vi "motor control proto.vi"(4 "minimal rot error":dbl=0.001, 6 "minimal error":dbl=0.001, 7 "motor link":enum16{"平移", "旋转", "压电控制"}(ring), 8 "error in (no error)":errorcluster caption="错误输入（无错误）", 9 "rotation num":dbl, 10 "target position":dbl=0.2 min=0.2 max=25.0 step=0.002) -> (0 "error out":errorcluster caption="错误输出", 1 "rotaion":dbl, 2 "position":dbl)   [LabVIEW 2017]
doc: "该模板用于创建子VI。"
uses:
  motor control.ctl
panel:
  out "Position":dbl[](array[numeric]) format="%.6f"
  in  "obj error":dbl=0.001
  out "objective":dbl min=0.0 max=250.0
  in  "target objective":dbl min=0.0 max=250.0
  in  "USB SET for E709":cluster{"S/N":string, "USB Search?":bool}={"S/N"="", "USB Search?"=TRUE}
  in  "RON settings 2":T1={"RON Affected axes"=[], "Reference mode"=[], "Check FRF?"=TRUE}
  in  "RON settings":T1={"RON Affected axes"=[], "Reference mode"=[], "Check FRF?"=TRUE}
  in  "DaisyChain settings for rotation":T2={"Register DC"=FALSE, "DaisyChain Search?"=TRUE, "Device ID"=2}
  in  "USB settings for rotation":cluster{"S/N":string, "USB Search?":bool}={"S/N"="0135500392", "USB Search?"=FALSE}
  in  "DaisyChain setting for move":T2={"Register DC"=FALSE, "DaisyChain Search?"=TRUE, "Device ID"=1}
  in  "USB setting for move":cluster{"S/N":string, "USB Search?":bool}={"S/N"="0135500392", "USB Search?"=FALSE}
  in  "断开通讯":bool
  in  "motor control":T3={"System no."=1, "Conn. \nAxes"=[], "当前数值"=[]} {"System no." min=1 step=1}
  # "parameter set"
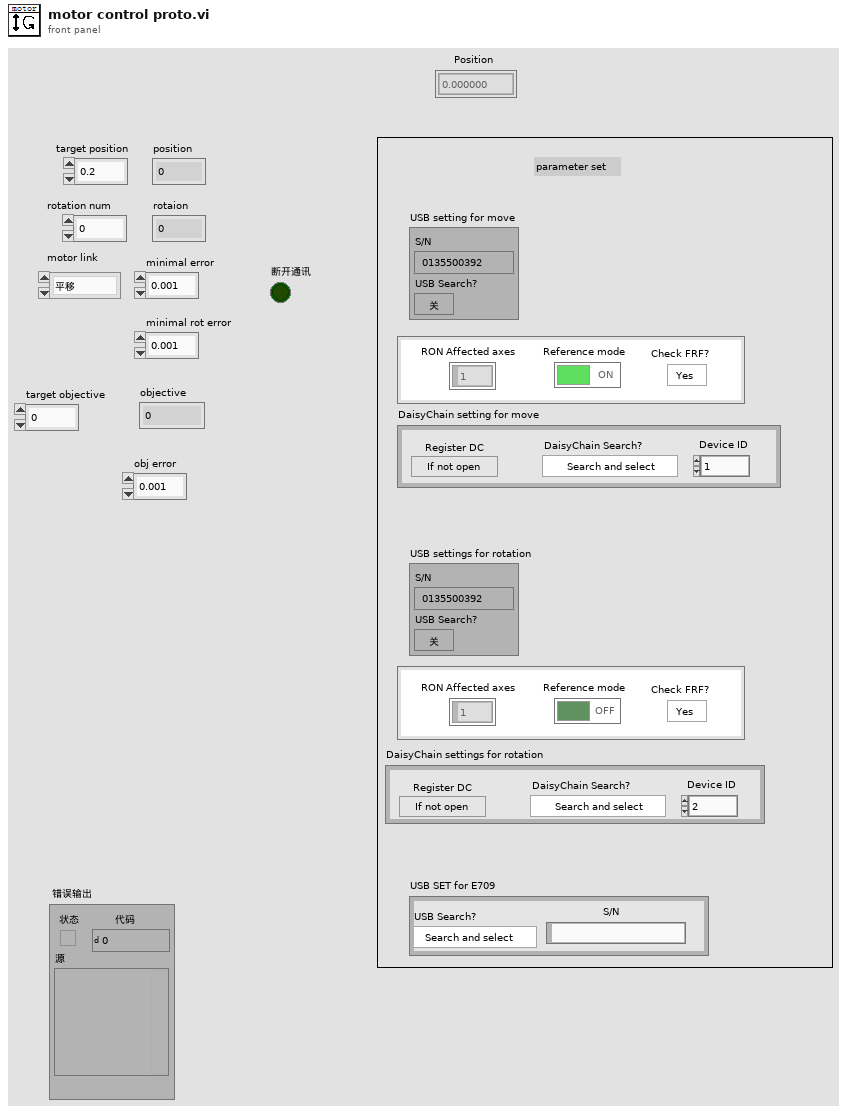
[diagram p1: front panel]
types:
  T1 = cluster{"RON Affected axes":string[], "Reference mode":bool[], "Check FRF?":bool}
  T2 = cluster{"Register DC":bool, "DaisyChain Search?":bool, "Device ID":i32}
  T3 = typedef "motor control.ctl" = cluster{"System no.":i32, "Conn. \nAxes":string[], "当前数值":dbl[]}
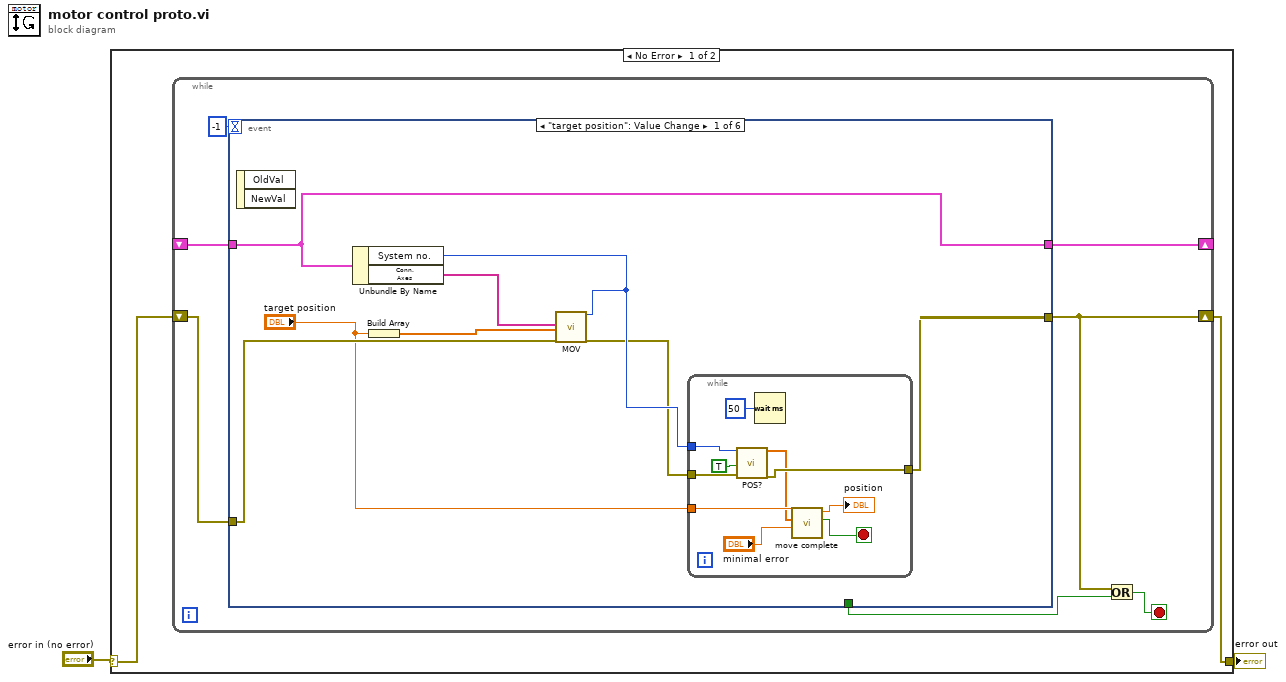
[diagram p0: block diagram]
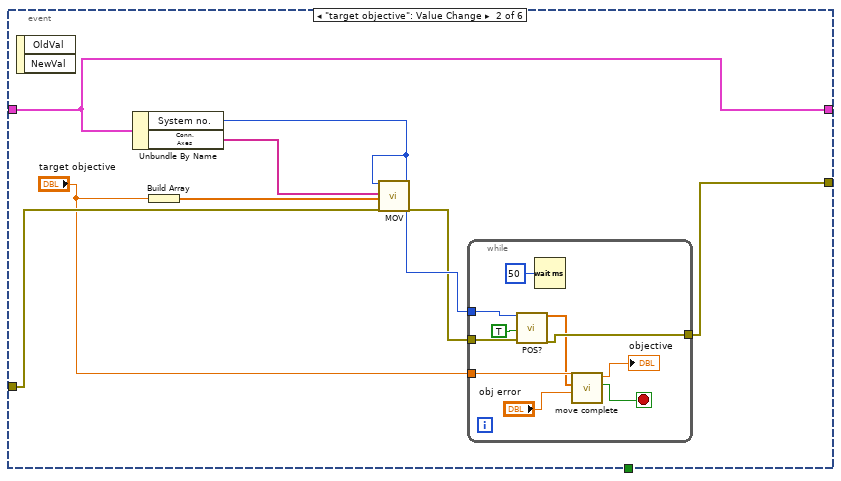
[diagram p2: hidden frame]
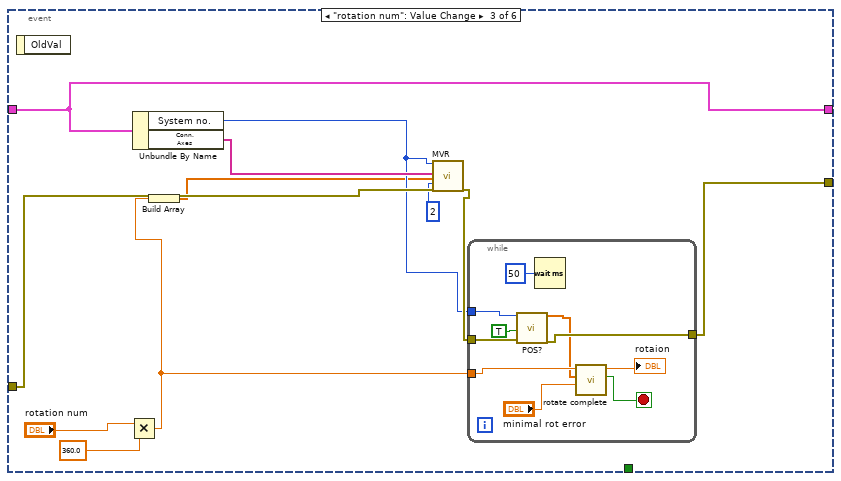
[diagram p3: hidden frame]
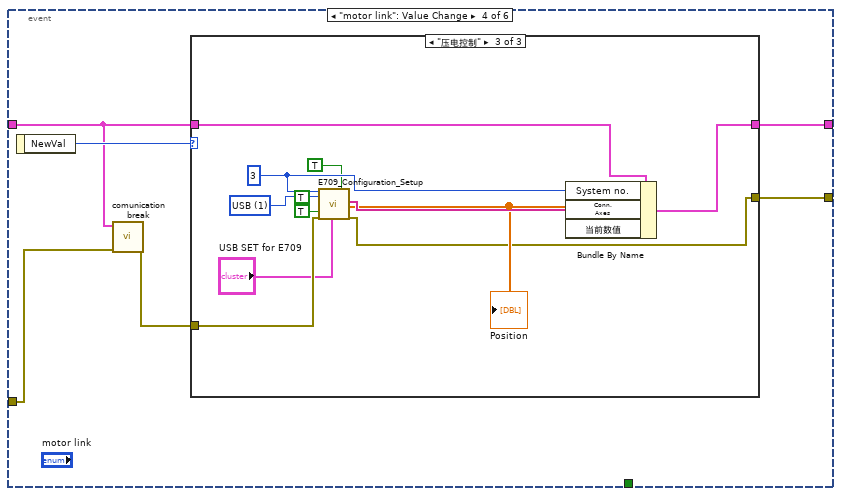
[diagram p4: hidden frame]
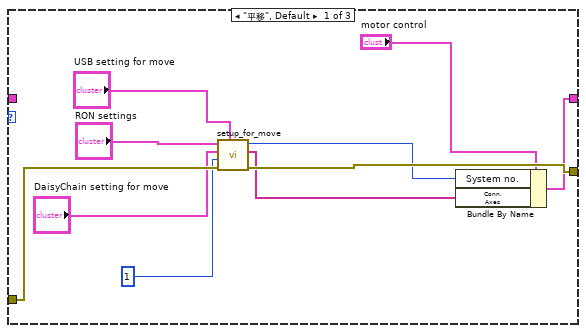
[diagram p5: hidden frame]
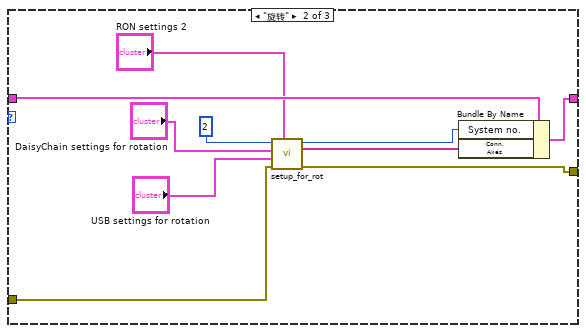
[diagram p6: hidden frame]
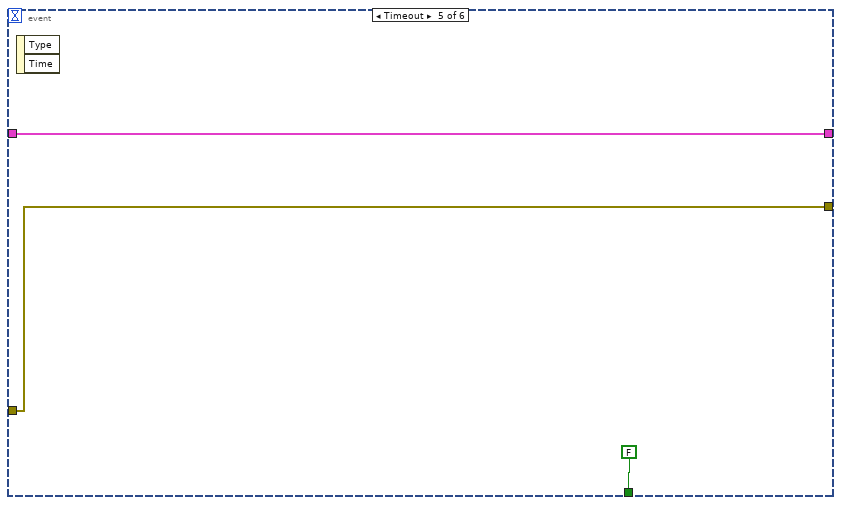
[diagram p7: hidden frame]
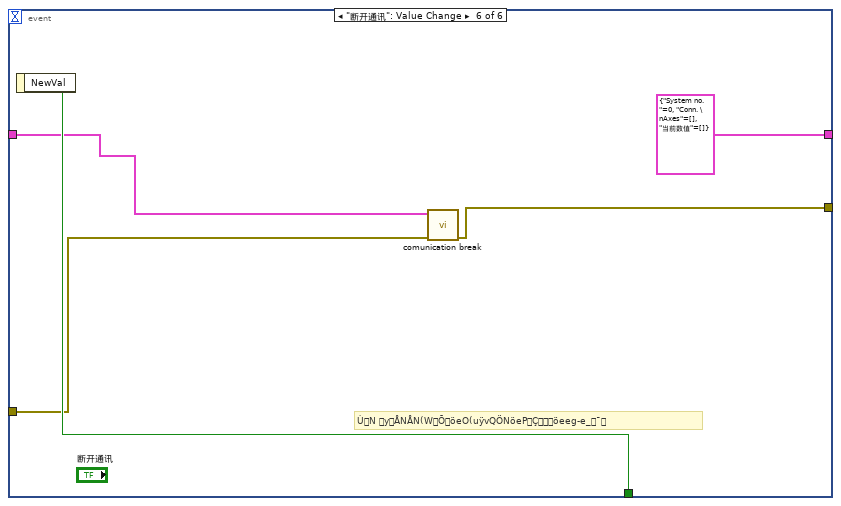
[diagram p8: hidden frame]
diagram:
  n1 = case shown="No Error" "error in (no error)" {
    selector: "error in (no error)" -> [w3 w115]
    tunnel: [w4 w115] -> w1
    frame No Error {
      n2 = while {
        shift-right: [w6] -> w4
        shift-left: w3 -> [w9]
        shift-right: [w11] -> _
        shift-left: _ -> [w10]
        stop <- w5 stop-if-true
        n3 = event shown="[0] \"target position\": Value Change" {
          selector: _ -> [_ _ _ _ _ _]
          dyn-events: _ -> [_ _ _ _ _ _]
          timeout: -1 -> [_ _ _ _ _ _]
          tunnel: [w13 w31 w57 w74 w107 w111] -> w6
          tunnel: w9 -> [w18 w36 w53 w71 w107 w112]
          tunnel: [w17 w35 w58 w73 w109 T3 {"System no."=0, "Conn. \nAxes"=[], "当前数值"=[]} ("motor control 2")] -> w11
          tunnel: w10 -> [w17 w35 w58 w69 w109 w113]
          tunnel: [_ _ _ _ FALSE ("NewVal") w114] -> w7
          event "target position": Value Change {
            n4 = event-data() -> ()  [unwired: 1 in, 2 out]
            n5 = Unbundle By Name(w17) -> ("System no."=w16:i32, "Conn. \nAxes"=w19:string[])
            n6 = Build Array("target position") -> (w14:dbl[])
            n7 = call "MOV.vi"("System no."=w16, "Axes to move"=w19, "Position values"=w14, "error in"=w18) -> ("error out"=w15:errorcluster)  [unwired: 15 in]
            n8 = while {
              tunnel: w16 -> [w29]
              tunnel: w15 -> [w27]
              tunnel: [w26] -> w13
              tunnel: "target position" -> [w23]
              stop <- w20 stop-if-true
              n9 = call "POS?.vi"("System no."=w29, "All axes?"=TRUE, "error in"=w27) -> ("Position"=w22:dbl[], "error out"=w26:errorcluster)  [unwired: 15 in]
              n10 = Wait (ms)(milliseconds to wait=u32 50 ("等待时间（毫秒）")) -> ()  [unwired: 1 out]
              n11 = call "move complete.vi"("minimal error"="minimal error", "Position"=w22, "target position"=w23) -> (2:w20:bool, "position output"=→"position":dbl)  [unwired: 6 in, 1 out]
            }
          }
          event "target objective": Value Change {
            n12 = event-data() -> ()  [unwired: 1 in, 2 out]
            n13 = Unbundle By Name(w35) -> ("System no."=w34:i32, "Conn. \nAxes"=w37:string[])
            n14 = Build Array("target objective") -> (w32:dbl[])
            n15 = call "MOV.vi"("System no."=w34, "Axes to move"=w37, "Position values"=w32, "error in"=w36) -> ("error out"=w33:errorcluster)  [unwired: 15 in]
            n16 = while {
              tunnel: w34 -> [w47]
              tunnel: w33 -> [w45]
              tunnel: [w44] -> w31
              tunnel: "target objective" -> [w41]
              stop <- w39 stop-if-true
              n17 = call "POS?.vi"("System no."=w47, "All axes?"=TRUE, "error in"=w45) -> ("Position"=w40:dbl[], "error out"=w44:errorcluster)  [unwired: 15 in]
              n18 = Wait (ms)(milliseconds to wait=u32 50 ("等待时间（毫秒）")) -> ()  [unwired: 1 out]
              n19 = call "move complete.vi"("minimal error"="obj error", "Position"=w40, "target position"=w41) -> (2:w39:bool, "position output"=→"objective":dbl)  [unwired: 6 in, 1 out]
            }
          }
          event "rotation num": Value Change {
            n20 = event-data() -> ()  [unwired: 1 in, 1 out]
            n21 = Multiply(x="rotation num", y=360.0) -> (x*y=w54:dbl)
            n22 = Unbundle By Name(w58) -> ("System no."=w50:i32, "Conn. \nAxes"=w51:string[])
            n23 = Build Array(w54) -> (w49:dbl[])
            n24 = call "MVR.vi"("System no."=w50, "Axes to move"=w51, "Position values"=w49, "No.of digits"=i16 2, "error in"=w53) -> ("error out"=w52:errorcluster)  [unwired: 14 in]
            n25 = while {
              tunnel: w50 -> [w68]
              tunnel: w52 -> [w66]
              tunnel: [w65] -> w57
              tunnel: w54 -> [w63]
              stop <- w60 stop-if-true
              n26 = call "POS?.vi"("System no."=w68, "All axes?"=TRUE, "error in"=w66) -> ("Position"=w62:dbl[], "error out"=w65:errorcluster)  [unwired: 15 in]
              n27 = Wait (ms)(milliseconds to wait=u32 50 ("等待时间（毫秒）")) -> ()  [unwired: 1 out]
              n28 = call "rotate complete.vi"("minimal error"="minimal rot error", "current rotation"=w62, "target rotation"=w63) -> ("rot complete"=w60:bool, "rotation number"=→"rotaion":dbl)  [unwired: 6 in, 1 out]
            }
          }
          event "motor link": Value Change {
            n29 = event-data() -> ("NewVal"=w72:enum16{"平移", "旋转", "压电控制"})  [unwired: 1 in]
            n30 = call "comunication break.vi"("错误输入（无错误）"=w71, "motor control输入"=w69) -> ("错误输出"=w70:errorcluster)  [unwired: 9 in]
            n31 = case shown="\"压电控制\"" w72 {
              tunnel: w70 -> [w84 w89 w105]
              tunnel: [w83 w88 w98] -> w74
              tunnel: [w79 w90 w99] -> w73
              tunnel: w69 -> [_ w87 w100]
              frame "平移", Default {
                n32 = call "setup_for_move.vi"("USB setting for move"="USB setting for move", "错误输入（无错误）"=w84, "System no.输入"=1 ("System no."), "DaisyChain setting for move"="DaisyChain setting for move", "RON settings"="RON settings") -> ("错误输出"=w83:errorcluster, "Conn. \nAxes"=w80:string[], "System no.输出"=w81:i32)  [unwired: 4 in]
                n33 = Bundle By Name(cluster="motor control", "System no."=w81, "Conn. \nAxes"=w80) -> (w79:T3)
              }
              frame "旋转" {
                n34 = call "setup_for_rot.vi"("RON settings"="RON settings 2", "错误输入（无错误）"=w89, "USB settings for rotation"="USB settings for rotation", "DaisyChain settings for rotation"="DaisyChain settings for rotation", "System no.输入"=2 ("System no. 2")) -> ("错误输出"=w88:errorcluster, "Conn. \nAxes"=w93:string[], "System no. 3"=w94:i32)  [unwired: 4 in]
                n35 = Bundle By Name(cluster=w87, "System no."=w94, "Conn. \nAxes"=w93) -> (w90:T3)
              }
              frame "压电控制" {
                w104 = u16 1 items=["RS232", "USB"] ("Interface")
                w103 = 3 ("System no.")
                n36 = call "E709_Configuration_Setup.vi"("System no."=w103, "Interface"=w104, "Change servo status to ON?"=TRUE, "Perform autozero?"=TRUE, "error in"=w105, "USB settings"="USB SET for E709", "Move to middle?"=TRUE) -> ("Conn. \nAxis"=w102:string[], "Position"=w101:dbl[], "error out"=w98:errorcluster)  [unwired: 7 in, 3 out]
                "Position" <- w101
                n37 = Bundle By Name(cluster=w100, "System no."=w103, "Conn. \nAxes"=w102, "当前数值"=w101) -> (w99:T3)
              }
            }
          }
          event Timeout {
            n38 = event-data() -> ()  [unwired: 1 in, 2 out]
          }
          event "断开通讯": Value Change {
            # "ÙN\tyÅNÅN(WÕöeO(uÿvQÖNöePÇöeeg­e_¯"
            n39 = event-data() -> ("NewVal"=w114:bool)  [unwired: 1 in]
            n40 = call "comunication break.vi"("错误输入（无错误）"=w112, "motor control输入"=w113) -> ("错误输出"=w111:errorcluster)  [unwired: 9 in]
          }
        }
        n41 = Or(x=w6, y=w7) -> (x .or. y?=w5:bool)
      }
    }
    frame Error {
    }
  }
  "error out" <- w1
